vi "Read Values.vi"(8 "error in (no error)":errorcluster, 11 "Simulated Scope in":refnum<class "Simulated Scope.lvclass">) -> (0 "error out":errorcluster, 2 "Values":dbl[](array[numeric]), 3 "Simulated Scope out":refnum<class "Simulated Scope.lvclass">)   [LabVIEW 2020, in "Simulated Scope.lvlib" / "Simulated Scope.lvclass"]
uses:
  Simulated Scope.lvclass
  Simulated Scope.lvclass/Simulated Scope.ctl
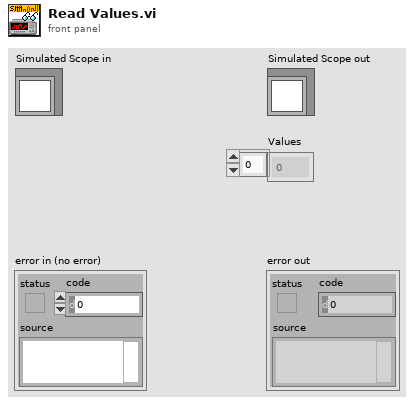
[diagram p1: front panel]
types:
  T1 = typedef "Simulated Scope.lvlib/Simulated Scope.lvclass/Ref Data.ctl" = cluster{"Sim Queue Name":string, "Waveform Queue":refnum<queue>}
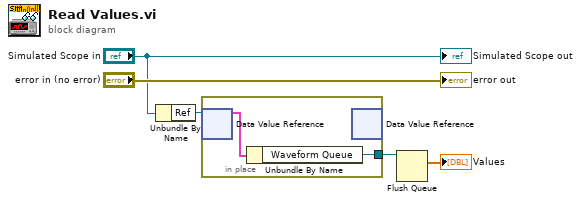
[diagram p0: block diagram]
diagram:
  n1 = Unbundle By Name("Simulated Scope in") -> ("Ref"=w4:refnum<data-value>)
  n2 = in-place {
    in-place-border: [w6] -> w2
    n3 = in-place-dvr #1(w4) -> (w7:T1)  [unwired: 1 out]
    n4 = Unbundle By Name(w7) -> ("Waveform Queue"=w6:refnum<queue>)
    n5 = in-place-dvr #1() -> ()  [unwired: 1 in, 2 out]
  }
  n6 = Flush Queue(queue=w2) -> (remaining elements=→"Values":dbl[])  [unwired: 1 in, 2 out]
  "error out" <- "error in (no error)"
  "Simulated Scope out" <- "Simulated Scope in"
